vi "SmallestAngle.vi"(10 "Angle B":dbl, 11 "Angle A":dbl) -> (3 "Smallest B to A":dbl)   [LabVIEW 2016]
doc: "Returns the smallest angle from A to B\n\nFor example, if A is 3600 and B is 0 it returns 0, because those are the same angle\n\nOutput is always in [-180, 180)"
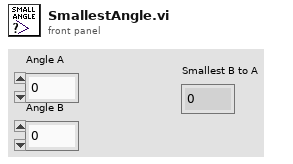
[diagram p1: front panel]
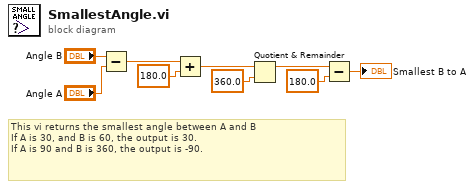
[diagram p0: block diagram]
diagram:
  # "This vi returns the smallest angle between A and B\nIf A is 30, and B is 60, the output is 30.\nIf A is 90 and B is 360, the output is -90."
  n1 = Subtract(x="Angle B", y="Angle A") -> (x-y=w9:dbl)
  n2 = Add(x=w9, y=180.0) -> (x+y=w7:dbl)
  n3 = Quotient & Remainder(x=w7, y=360.0) -> (x-y*floor(x/y)=w5:dbl)  [unwired: 1 out]
  n4 = Subtract(x=w5, y=180.0) -> (x-y=→"Smallest B to A":dbl)
